vi "FGV_Message Manager.vi"(8 "error in (no error)":errorcluster, 10 "Parameter":variant, 11 "Command":T2) -> (0 "error out":errorcluster, 2 "Parameter out":variant, 3 "UI to Controller Message":T1)   [LabVIEW 2012]
uses:
  DataType/FGV_Message Manager_Command.ctl
  DataType/Simulation Console_User Action.ctl
  DataType/Simulation Console_Command To UI.ctl
  DataType/Simulation Console_Controller Command.ctl
  DataType/Simulation Console_Data From UI.ctl
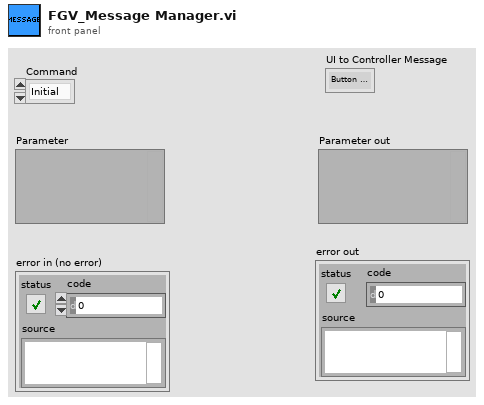
[diagram p1: front panel]
types:
  T1 = typedef "Simulation Console_User Action.ctl" = enum16{"Button Press", "Card Insert", "Card Remove", "Keypad Input"}
  T2 = typedef "FGV_Message Manager_Command.ctl" = enum16{"Initial", "Close", "SendMessage", "SendButton", "DisableUI", "ClearKeypad", "ReturnCard", "RecieveUserInput"}
  T3 = typedef "Simulation Console_Command To UI.ctl" = cluster{"Command":T4, "Parameter":variant}
  T4 = typedef "Simulation Console_Controller Command.ctl" = enum16{"Show Message", "Return Card", "Stop", "Show Menu", "Clear Keypad", "Disable UI Element"}
  T5 = typedef "Simulation Console_Data From UI.ctl" = cluster{"UI to Controller Message":T1, "Parameter":variant}
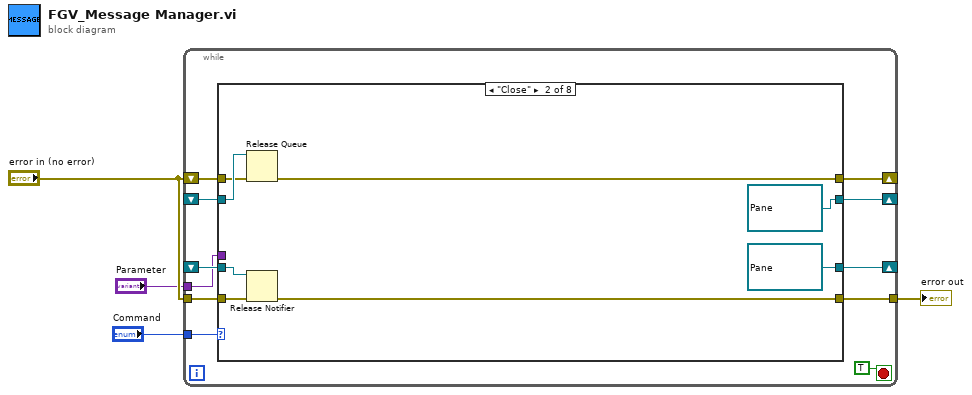
[diagram p0: block diagram]
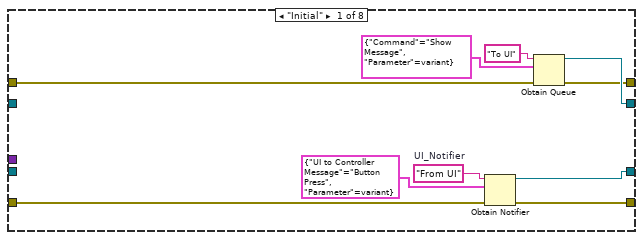
[diagram p2: hidden frame]
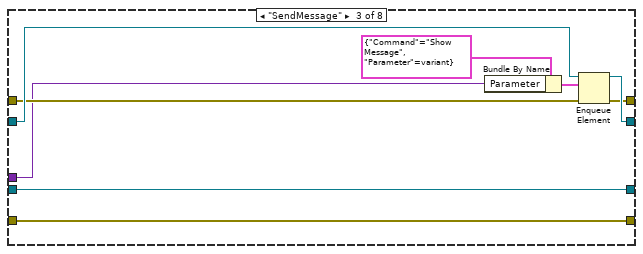
[diagram p3: hidden frame]
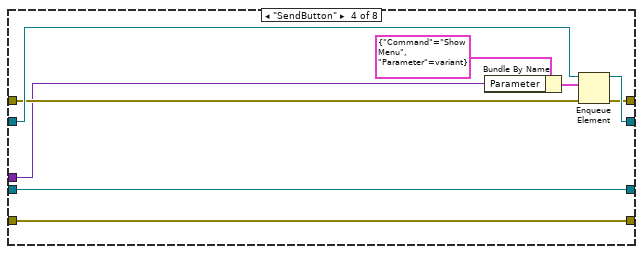
[diagram p4: hidden frame]
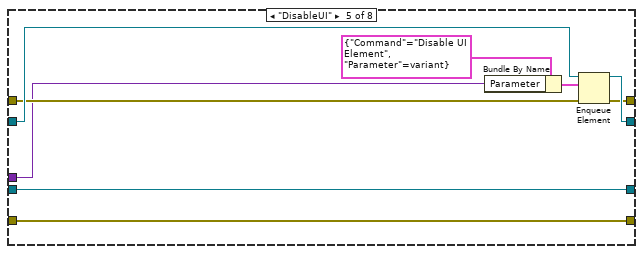
[diagram p5: hidden frame]
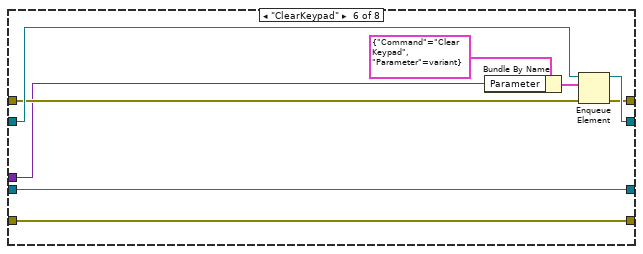
[diagram p6: hidden frame]
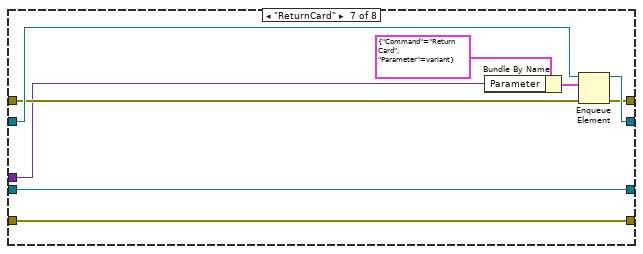
[diagram p7: hidden frame]
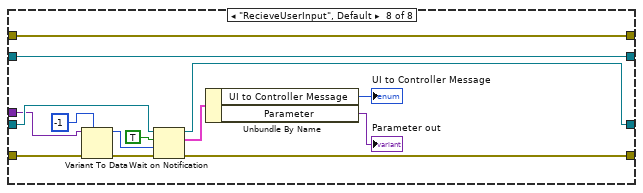
[diagram p8: hidden frame]
diagram:
  n1 = while {
    tunnel: "Command" -> [w14]
    tunnel: "error in (no error)" -> [w13]
    tunnel: [w12] -> w3
    shift-right: [w11] -> _
    shift-left: "error in (no error)" -> [w10]
    shift-right: [w9] -> _
    shift-left: _ -> [w8]
    shift-right: [w7] -> _
    shift-left: _ -> [w6]
    tunnel: "Parameter" -> [w5]
    stop <- TRUE ("stop") stop-if-true
    n2 = case shown="\"Close\"" w14 {
      tunnel: [w21 refnum<queue> refnum ("queue out") w40 w49 w58 w67 w76 w92] -> w9
      tunnel: [w20 refnum<notifier> refnum ("notifier out") w37 w46 w55 w64 w73 w87] -> w7
      tunnel: w13 -> [w19 w29 w41 w50 w59 w68 w77 w80]
      tunnel: [w18 w28 w41 w50 w59 w68 w77 w90] -> w12
      tunnel: [w17 w31 w38 w47 w56 w65 w74 w91] -> w11
      tunnel: w10 -> [w16 w32 w39 w48 w57 w66 w75 w91]
      tunnel: w8 -> [_ w33 w42 w51 w60 w69 w78 w92]
      tunnel: w6 -> [_ w30 w37 w46 w55 w64 w73 w89]
      tunnel: w5 -> [_ _ w34 w43 w52 w61 w70 w83]
      frame "Initial" {
        w25 = "From UI"  # UI_Notifier
        n3 = Obtain Notifier(name (unnamed)=w25, notification data type=T5 {"UI to Controller Message"=enum."Button Press", "Parameter"=variant}, error in (no error)=w19) -> (notifier out=w20:refnum<notifier>, error out=w18:errorcluster)  [unwired: 1 in, 1 out]
        n4 = Obtain Queue(name (unnamed)="To UI", element data type=T3 {"Command"=enum."Show Message", "Parameter"=variant}, error in (no error)=w16) -> (queue out=w21:refnum<queue>, error out=w17:errorcluster)  [unwired: 2 in, 1 out]
      }
      frame "Close" {
        n5 = Release Queue(queue=w33, error in (no error)=w32) -> (error out=w31:errorcluster)  [unwired: 1 in, 2 out]
        n6 = Release Notifier(notifier=w30, error in (no error)=w29) -> (error out=w28:errorcluster)  [unwired: 1 in, 2 out]
      }
      frame "SendMessage" {
        n7 = Bundle By Name(cluster=T3 {"Command"=enum."Show Message", "Parameter"=variant} ("element"), "Parameter"=w34) -> (w35:T3)
        n8 = Enqueue Element(queue=w42, element=w35, error in (no error)=w39) -> (queue out=w40:refnum<queue>, error out=w38:errorcluster)  [unwired: 1 in, 1 out]
      }
      frame "SendButton" {
        n9 = Bundle By Name(cluster=T3 {"Command"=enum."Show Menu", "Parameter"=variant} ("element"), "Parameter"=w43) -> (w44:T3)
        n10 = Enqueue Element(queue=w51, element=w44, error in (no error)=w48) -> (queue out=w49:refnum<queue>, error out=w47:errorcluster)  [unwired: 1 in, 1 out]
      }
      frame "DisableUI" {
        n11 = Bundle By Name(cluster=T3 {"Command"=enum."Disable UI Element", "Parameter"=variant} ("element"), "Parameter"=w52) -> (w53:T3)
        n12 = Enqueue Element(queue=w60, element=w53, error in (no error)=w57) -> (queue out=w58:refnum<queue>, error out=w56:errorcluster)  [unwired: 1 in, 1 out]
      }
      frame "ClearKeypad" {
        n13 = Bundle By Name(cluster=T3 {"Command"=enum."Clear Keypad", "Parameter"=variant} ("element"), "Parameter"=w61) -> (w62:T3)
        n14 = Enqueue Element(queue=w69, element=w62, error in (no error)=w66) -> (queue out=w67:refnum<queue>, error out=w65:errorcluster)  [unwired: 1 in, 1 out]
      }
      frame "ReturnCard" {
        n15 = Bundle By Name(cluster=T3 {"Command"=enum."Return Card", "Parameter"=variant} ("element"), "Parameter"=w70) -> (w71:T3)
        n16 = Enqueue Element(queue=w78, element=w71, error in (no error)=w75) -> (queue out=w76:refnum<queue>, error out=w74:errorcluster)  [unwired: 1 in, 1 out]
      }
      frame "RecieveUserInput", Default {
        n17 = Variant To Data(error in=w80, type=-1 ("timeout in ms (-1)"), Variant=w83) -> (data=w81:i32, error out=w79:errorcluster)
        n18 = Wait on Notification(notifier=w89, ignore previous (F)=TRUE, timeout in ms (-1)=w81, error in (no error)=w79) -> (notifier out=w87:refnum<notifier>, notification=w86:T5, error out=w90:errorcluster)  [unwired: 1 out]
        n19 = Unbundle By Name(w86) -> ("UI to Controller Message"=→"UI to Controller Message":T1, "Parameter"=→"Parameter out":variant)
      }
    }
  }
  "error out" <- w3
